vi "GetActualDepsListPath.vi"(8 "error in (no error)":errorcluster) -> (0 "error out":errorcluster, 3 "ActualDepsListPath":path)   [LabVIEW 2019, in "DepsWatch.lvlib"]
uses:
  DepsWatch.lvlib
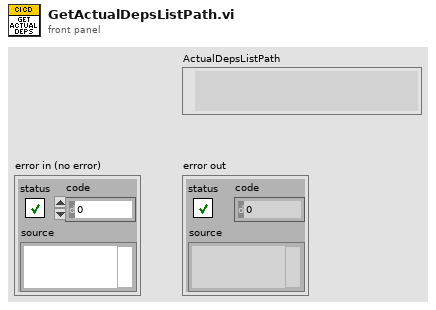
[diagram p1: front panel]
types:
  T1 = typedef "DepsWatch.lvlib/CICDPathConfigs.ctl" = cluster{"GlobalIncludePaths":path[], "GlobalExcludePaths":path[], "BuildSpecsIncludePaths":path[], "ActualDepsIncludePaths":path[], "WorkspacePath":path, "SourceFolderPaths":path[], "ChangedFilesLogpaths":map{string, path}}
  T2 = enum16{"open", "replace", "create", "open or create", "replace or create", "replace or create with confirmation"}
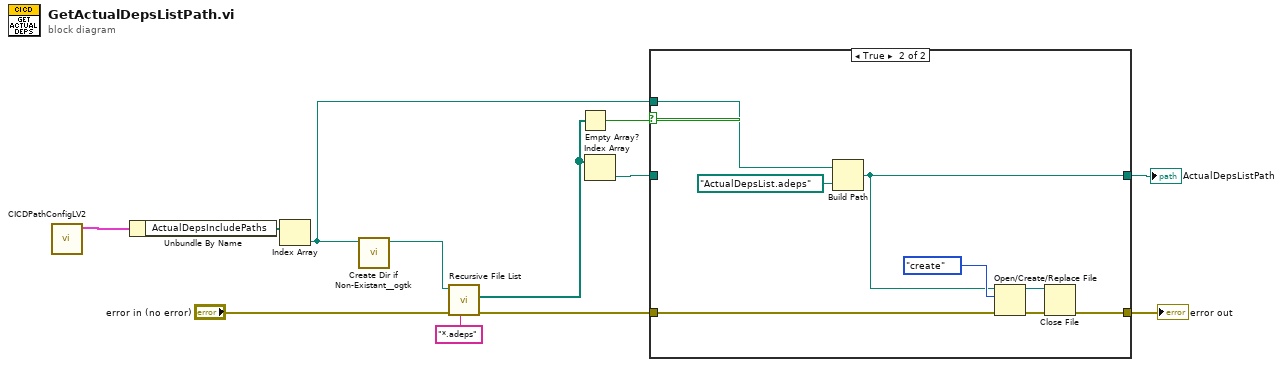
[diagram p0: block diagram]
diagram:
  n1 = call "CICDPathConfigLV2.vi"() -> ("CICD Path Config Out"=w10:T1)  [unwired: 11 in]
  n2 = Unbundle By Name(w10) -> ("ActualDepsIncludePaths"=w11:path[])
  n3 = Index Array(array=w11) -> (element=w7:path)  [unwired: 1 in]
  n4 = call <userlib>:"Create Dir if Non-Existant__ogtk.vi"("Directory Path"=w7) -> ("dup Directory Path"=w1:path)  [unwired: 8 in, 2 out]
  n5 = call <vilib>:"Recursive File List.vi"("pattern"="*.adeps", "error in (no error)"="error in (no error)", "Folder Path"=w1) -> ("error out"=w3:errorcluster, "All Files in Dir"=w9:path[])  [unwired: 4 in, 3 out]
  n6 = Empty Array?(array=w9) -> (empty?=w8:bool)
  n7 = Index Array(array=w9) -> (element=w6:path)  [unwired: 1 in]
  n8 = case shown="True" w8 {
    tunnel: w7 -> [_ w22]
    tunnel: w6 -> [w14 _]
    tunnel: [w14 w17] -> w5
    tunnel: [w13 w16] -> w2
    tunnel: w3 -> [w13 w15]
    frame False {
    }
    frame True {
      n9 = Build Path(base path=w22, name or relative path=path "ActualDepsList.adeps") -> (appended path=w17:path)
      n10 = Open/Create/Replace File(file path (use dialog)=w17, error in=w15, operation (0:open)=T2."create") -> (refnum out=w20:refnum<file>, error out=w19:errorcluster)  [unwired: 3 in, 1 out]
      n11 = Close File(refnum=w20, error in=w19) -> (error out=w16:errorcluster)  [unwired: 1 out]
    }
  }
  "ActualDepsListPath" <- w5
  "error out" <- w2
